vi "Get Sampling Rate.vi"(8 "error in (no error)":errorcluster, 11 "EPU452 in":refnum<class "EPU452.lvclass">) -> (0 "error out":errorcluster, 1 "Sampling Rate (Hz)":dbl, 2 "Response":string, 3 "EPU452 out":refnum<class "EPU452.lvclass">)   [LabVIEW 2018, in "EPU452.lvclass"]
uses:
  EPU452.lvclass
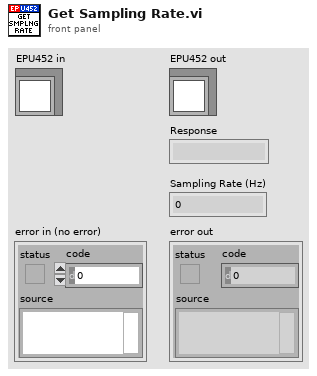
[diagram p1: front panel]
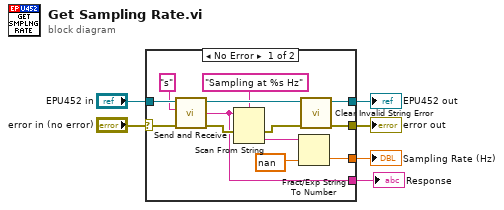
[diagram p0: block diagram]
diagram:
  n1 = case shown="No Error" "error in (no error)" {
    selector: "error in (no error)" -> [w18 w21]
    tunnel: [w9 w21] -> w5
    tunnel: [w15 w20] -> w3
    tunnel: "EPU452 in" -> [w19 w20]
    tunnel: [w8 _] -> w2
    tunnel: [w7 _] -> w1
    frame No Error {
      n2 = call "Send and Receive.vi"("error in (no error)"=w18, "Command"="s", "EPU452 in"=w19) -> ("error out"=w14:errorcluster, "Response"=w7:string, "EPU452 out"=w16:refnum<class "EPU452.lvclass">)  [unwired: 6 in]
      n3 = Scan From String(format string="Sampling at %s Hz", input string=w7, error in=w14) -> (error out=w10:errorcluster, output 1=w11:string)  [unwired: 2 in, 2 out]
      n4 = Fract/Exp String To Number(string=w11, default (0 dbl)=nan ("default (0 DBL)")) -> (number=w8:dbl)  [unwired: 2 in, 1 out]
      n5 = call "Clear Invalid String Error.vi"("error in (no error)"=w10, "EPU452 in"=w16) -> ("error out"=w9:errorcluster, "EPU452 out"=w15:refnum<class "EPU452.lvclass">)  [unwired: 8 in]
    }
    frame Error {
    }
  }
  "error out" <- w5
  "EPU452 out" <- w3
  "Sampling Rate (Hz)" <- w2
  "Response" <- w1
